vi "my DWDT Boolean Array to Digital.vi"(5 "compress data (T)":bool, 6 "t0":timestamp, 8 "error in (no error)":errorcluster, 9 "mode":enum16{"LSB First", "MSB First"}(ring), 10 "sample rate":dbl=1000.0 format="%#_6p", 11 "boolean array":bool[][](array[boolean])) -> (0 "error out":errorcluster, 3 "digital waveform":digitalwaveform(waveform)={"t0"=timestamp(0 s since 1904-01-01), "dt"=0.0, "Y"={"transitions"=[], "data"=[]}, "error"={"status"=FALSE, "code"=37421928, "source"=""}})   [LabVIEW 2013]
doc: "Converts a 2D Boolean array to a digital waveform or digital data. You must manually select the polymorphic instance you want to use."
panel:
  in  "Empty Digital WDT":digitalwaveform(waveform)={"t0"=timestamp(0 s since 1904-01-01), "dt"=0.0, "Y"={"transitions"=[], "data"=[]}, "error"={"status"=FALSE, "code"=37421928, "source"=""}}
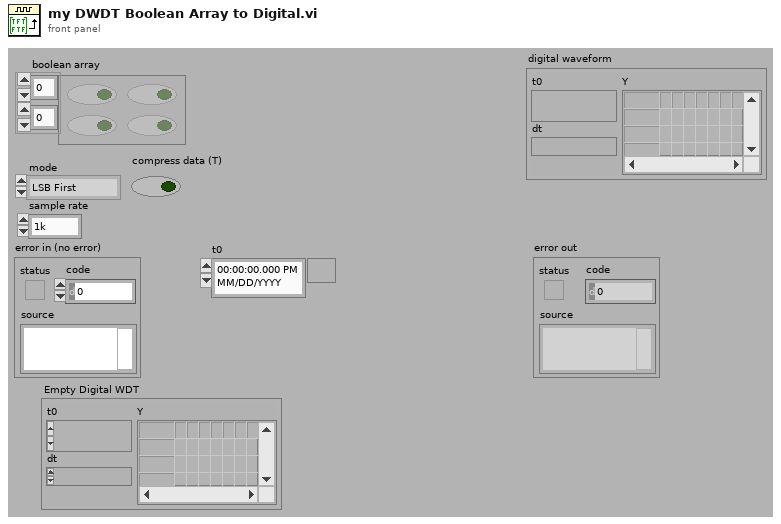
[diagram p1: front panel]
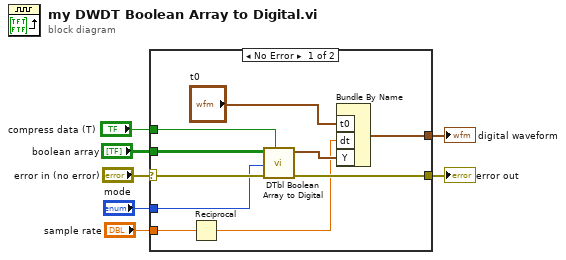
[diagram p0: block diagram]
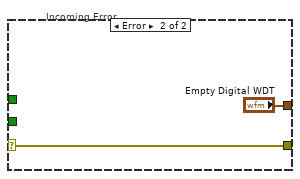
[diagram p2: hidden frame]
diagram:
  n1 = case shown="No Error" "error in (no error)" {
    selector: "error in (no error)" -> [w17 w19]
    tunnel: [w16 w19] -> w7
    tunnel: "boolean array" -> [w15 _]
    tunnel: [w13 "Empty Digital WDT"] -> w4
    tunnel: "mode" -> [w11 _]
    tunnel: "compress data (T)" -> [w10 _]
    tunnel: "sample rate" -> [w9 _]
    frame No Error {
      n2 = Reciprocal(x=w9) -> (1/x=w8:dbl)
      n3 = call <vilib>:"DTbl Boolean Array to Digital.vi"("compress data (F)"=w10, "error in (no error)"=w17, "mode"=w11, "boolean array"=w15) -> ("error out"=w16:errorcluster, "digital data"=w14:digitaldata)  [unwired: 6 in]
      n4 = Bundle By Name("t0"="t0", "dt"=w8, "Y"=w14) -> (w13:digitalwaveform)  [unwired: 1 in]
    }
    frame Error {
      # "Incoming Error"
    }
  }
  "digital waveform" <- w4
  "error out" <- w7
